vi "SPCDataCluster2TACAll&SysParPerModule.vi"(11 "SPCdata In":T3) -> (2 "User Input PerModules":T1={"sync_threshold"=-20.0, "sync_zc_level"=5.0, "sync_freq_div"=0, "cfd_limit_low"=0.0, "cfd_zc_level"=0.0} {"sync_freq_div" items=["1"=1, "2"=2, "4"=4]; "cfd_zc_level" min=-96 max=96 step=0.1 format="%#_3g"; "cfd_limit_low" min=-500 max=0 step=0.1 format="%#_3g"; "sync_zc_level" min=-96 max=96 step=0.1 format="%#_3g"; "sync_threshold" min=-500 max=-20 step=0.1 format="%#_3g"}, 3 "User Input AllModules":T2={"tac_range"=50.0, "tac_gain"=4, "tac_offset"=12.0, "tac_limit_high"=5.0, "tac_limit_low"=95.0, "collect_time"=0.1} {"tac_limit_high" min=0 max=100 step=0.1; "collect_time" min=1e-07 max=100000 step=0.001; "tac_offset" min=0 max=100 step=0.1; "tac_gain" min=1 max=15 step=1; "tac_range" format="%^#_6g"})   [LabVIEW 2023]
doc: "Only a small portion of all parameters in SPCData need adjustment in a specified measurement environment. \nThis VI transfers these data from the SPCData cluster into the UserInput AllModules and UserInput PerModules cluster.\nUse this VI to display the actual parameters accepted by the modules.\n\ninfo@becker-hickl.com"
uses:
  SPC_Wrappers/SPC_Controls/SPCdata.ctl
  Example_Controls/UserInput-AllModules.ctl
  Example_Controls/UserInput-PerModules.ctl
panel:
  # "CFD"
  # "(start)"
  # "SYNC"
  # "(stop)"
  # "threshold(LL)"
  # "zero cross(ZC)"
  # "TAC / Time Range"
  # "range"
  # "gain"
  # "offset"
  # "limit high"
  # "limit low"
  # "Collection Time"
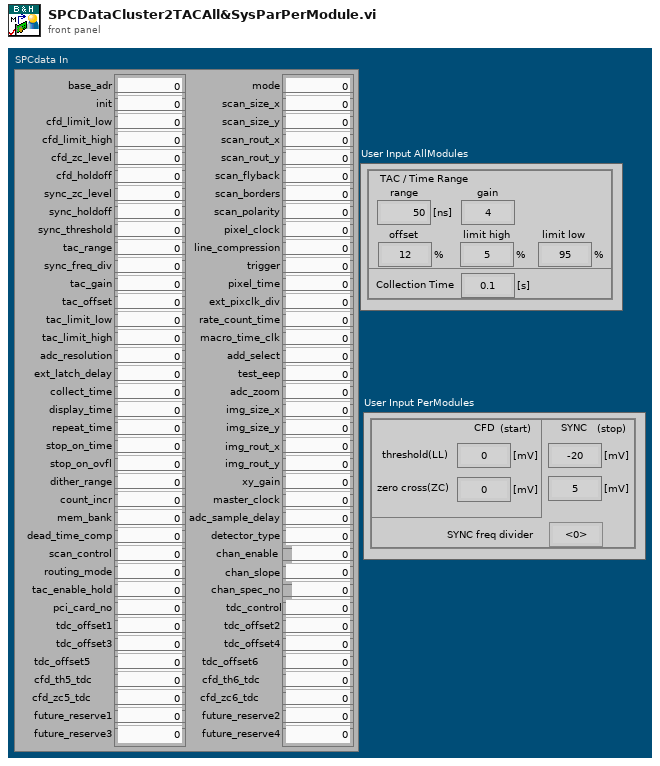
[diagram p1: front panel]
types:
  T1 = typedef "UserInput-PerModules.ctl" = cluster{"sync_threshold":sgl, "sync_zc_level":sgl, "sync_freq_div":i16, "cfd_limit_low":sgl, "cfd_zc_level":sgl}
  T2 = typedef "UserInput-AllModules.ctl" = cluster{"tac_range":sgl, "tac_gain":i16, "tac_offset":sgl, "tac_limit_high":sgl, "tac_limit_low":sgl, "collect_time":sgl}
  T3 = typedef "SPCdata.ctl" = cluster{"base_adr":u16, "init":i16, "cfd_limit_low":sgl, "cfd_limit_high":sgl, "cfd_zc_level":sgl, "cfd_holdoff":sgl, "sync_zc_level":sgl, "sync_holdoff":sgl, "sync_threshold":sgl, "tac_range":sgl, "sync_freq_div":i16, "tac_gain":i16, "tac_offset":sgl, "tac_limit_low":sgl, "tac_limit_high":sgl, "adc_resolution":i16, "ext_latch_delay":i16, "collect_time":sgl, "display_time":sgl, "repeat_time":sgl, "stop_on_time":i16, "stop_on_ovfl":i16, "dither_range":i16, "count_incr":i16, "mem_bank":i16, "dead_time_comp":i16, "scan_control":u16, "routing_mode":u16, "tac_enable_hold":sgl, "pci_card_no":i16, "mode":u16, "scan_size_x":u32, "scan_size_y":u32, "scan_rout_x":u32, "scan_rout_y":u32, "scan_flyback":u32, "scan_borders":u32, "scan_polarity":u16, "pixel_clock":u16, "line_compression":u16, "trigger":u16, "pixel_time":sgl, "ext_pixclk_div":u32, "rate_count_time":sgl, "macro_time_clk":i16, "add_select":i16, "test_eep":i16, "adc_zoom":i16, "img_size_x":u32, "img_size_y":u32, "img_rout_x":u32, "img_rout_y":u32, "xy_gain":i16, "master_clock":i16, "adc_sample_delay":i16, "detector_type":i16, "chan_enable":u32, "chan_slope":u32, "chan_spec_no":u32, "tdc_control":u32, "tdc_offset1":sgl, "tdc_offset2":sgl, "tdc_offset3":sgl, "tdc_offset4":sgl, "tdc_offset5":sgl, "tdc_offset6":sgl, "cfd_th5_tdc":sgl, "cfd_th6_tdc":sgl, "cfd_zc5_tdc":sgl, "cfd_zc6_tdc":sgl, "future_reserve1":u64, "future_reserve2":u64, "future_reserve3":u64, "future_reserve4":u64}
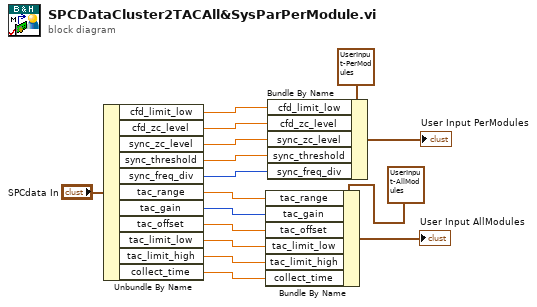
[diagram p0: block diagram]
diagram:
  n1 = Unbundle By Name("SPCdata In") -> ("cfd_limit_low"=w11:sgl, "cfd_zc_level"=w10:sgl, "sync_zc_level"=w9:sgl, "sync_threshold"=w8:sgl, "sync_freq_div"=w7:i16, "tac_range"=w6:sgl, "tac_gain"=w5:i16, "tac_offset"=w4:sgl, "tac_limit_low"=w3:sgl, "tac_limit_high"=w2:sgl, "collect_time"=w1:sgl)
  n2 = Bundle By Name(cluster=T2 {"tac_range"=50.0, "tac_gain"=4, "tac_offset"=12.0, "tac_limit_high"=5.0, "tac_limit_low"=95.0, "collect_time"=0.1} ("User Input AllModules"), "tac_range"=w6, "tac_gain"=w5, "tac_offset"=w4, "tac_limit_low"=w3, "tac_limit_high"=w2, "collect_time"=w1) -> (→"User Input AllModules":T2)
  n3 = Bundle By Name(cluster=T1 {"sync_threshold"=-123.0, "sync_zc_level"=5.0, "sync_freq_div"=0, "cfd_limit_low"=-80.0, "cfd_zc_level"=9.8} ("User Input PerModules"), "cfd_limit_low"=w11, "cfd_zc_level"=w10, "sync_zc_level"=w9, "sync_threshold"=w8, "sync_freq_div"=w7) -> (→"User Input PerModules":T1)
